vi "Write Self Attributes.vi"(7 "Actor in":refnum<class "Actor.lvclass">, 10 "Self Attributes":refnum<class "Attributes.lvclass">) -> (5 "Actor out":refnum<class "Actor.lvclass">)   [LabVIEW 2025, in "jettl.lvlib"]
uses:
  jettl.lvlib
  Attributes/Attributes.lvclass
  Actor/Actor.lvclass
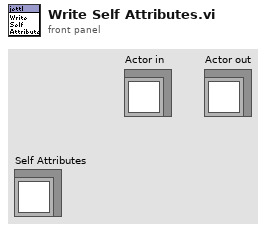
[diagram p1: front panel]
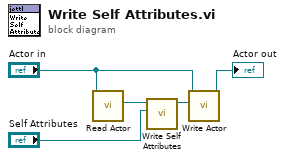
[diagram p0: block diagram]
diagram:
  n1 = call-dynamic "Read Actor.vi"("Actor in"="Actor in") -> ("Actor"=w5:refnum<class "Actor.lvclass">)  [unwired: 10 in]
  n2 = call-dynamic "Write Self Attributes.vi"("Self Attributes"="Self Attributes", "Actor in"=w5) -> ("Actor out"=w4:refnum<class "Actor.lvclass">)  [unwired: 9 in]
  n3 = call-dynamic "Write Actor.vi"("Actor"=w4, "Actor in"="Actor in") -> ("Actor out"=→"Actor out":refnum<class "Actor.lvclass">)  [unwired: 9 in]
